vi "Send Close.vi"(8 "error in (no error)":errorcluster, 11 "TCP Comm In":T1) -> (0 "error out":errorcluster, 3 "TCP Comm":T1)   [LabVIEW 2020, in "TinyTCP.lvlib"]
uses:
  TinyTCP.lvlib
  State.ctl
  Ref Data.ctl
  Instance.ctl
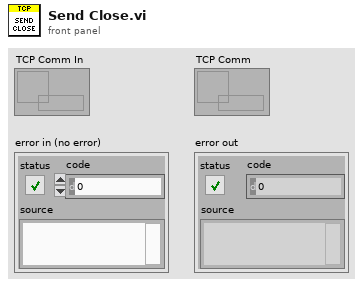
[diagram p1: front panel]
types:
  T1 = typedef "TinyTCP.lvlib/Instance.ctl" = refnum<data-value>
  T2 = typedef "TinyTCP.lvlib/Ref Data.ctl" = cluster{"TCP":refnum<k5>, "State":T3, "Server":bool, "Host":string, "Port":u16, "Listener":refnum<k5>, "Start":bool, "Disconnect":bool, "TCP Valid":bool, "TLS Enabled":bool, "Immutable TLS":refnum<k36>, "Certificate DN":string}
  T3 = typedef "TinyTCP.lvlib/State.ctl" = enum16{"Idle", "Starting", "Connecting", "Connected", "Disconnecting", "Stopped"}
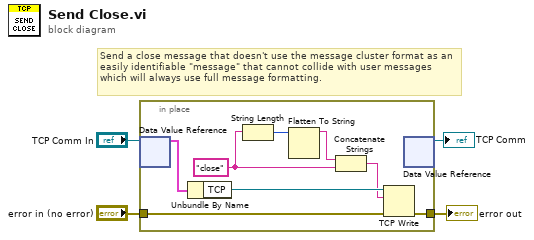
[diagram p0: block diagram]
diagram:
  # "Send a close message that doesn't use the message cluster format as an easily identifiable \"message\" that cannot collide with user messages which will always use full message formatting."
  n1 = in-place {
    in-place-border: "error in (no error)" -> [w12]
    in-place-border: [w5] -> w2
    w8 = "close" ("data in")
    n2 = in-place-dvr #1("TCP Comm In") -> (w11:T2)  [unwired: 1 out]
    n3 = Unbundle By Name(w11) -> ("TCP"=w10:refnum<k5>)
    n4 = String Length(string=w8) -> (length=w9:i32)
    n5 = Flatten To String(anything=w9) -> (data string=w7:string)  [unwired: 3 in, 2 out]
    n6 = Concatenate Strings(w7, w8) -> (w6:string)
    n7 = TCP Write(connection ID=w10, data in=w6, error in (no error)=w12) -> (error out=w5:errorcluster)  [unwired: 1 in, 2 out]
    n8 = in-place-dvr #1() -> (→"TCP Comm":T1)  [unwired: 1 in, 1 out]
  }
  "error out" <- w2
